vi "ShopTable.vi"(4 "食品信息":cluster{"ID":dbl, "食品名称":string, "价格":dbl}, 6 "枚举":enum16{"保存", "获取", "清空", "插入", "删除", "查询"}(ring)) -> (0 "Exist?":bool, 2 "食品信息 2":cluster{"ID":dbl, "食品名称":string, "价格":dbl}, 3 "数组":cluster{"ID":dbl, "食品名称":string, "价格":dbl}[](array[cluster]))   [LabVIEW 2013, in "InfoTable.lvclass"]
uses:
  InfoTable.lvclass
  FoodBase.lvclass
panel:
  in  "第一次？":bool
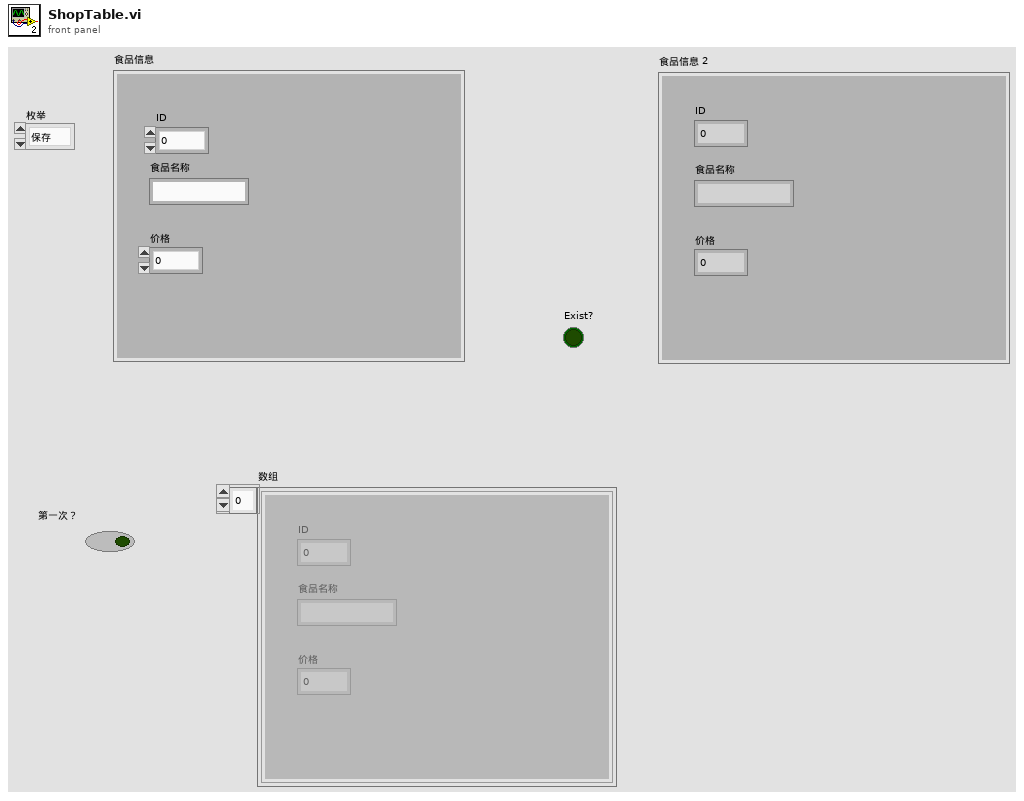
[diagram p1: front panel]
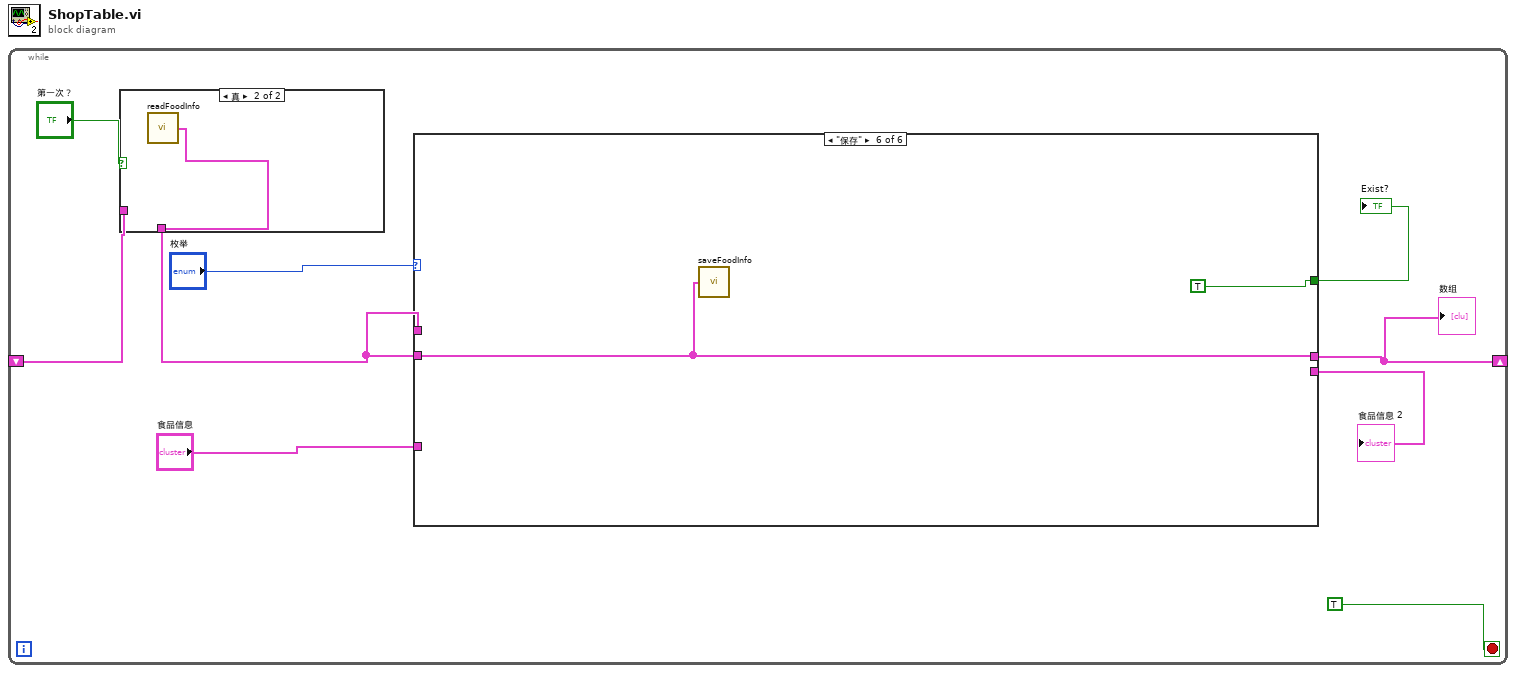
[diagram p0: block diagram]
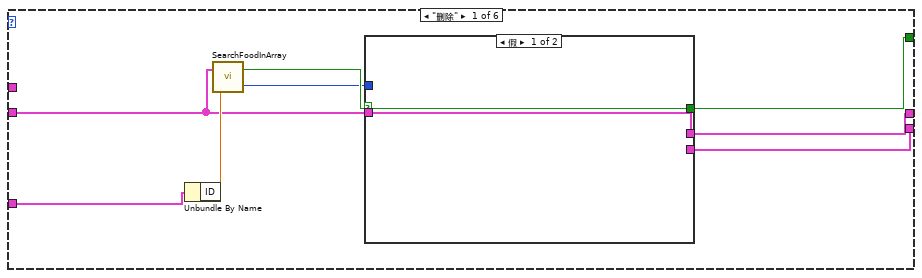
[diagram p3: hidden frame]
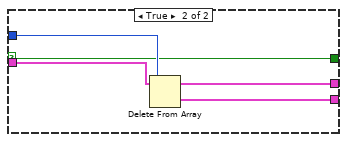
[diagram p4: hidden frame]
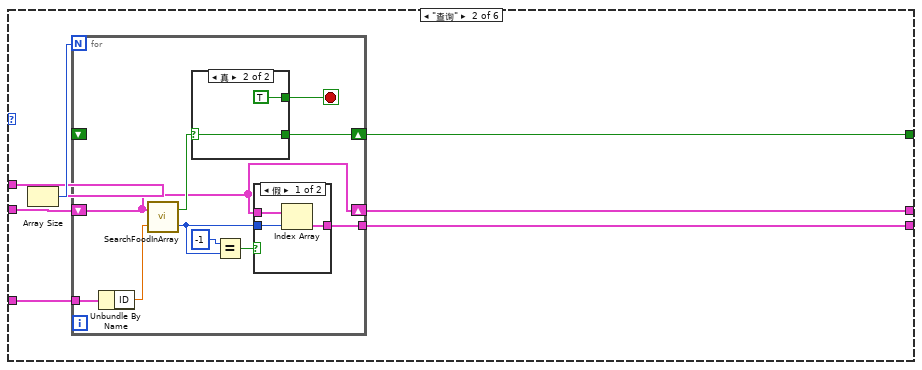
[diagram p5: hidden frame]
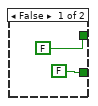
[diagram p7: hidden frame]
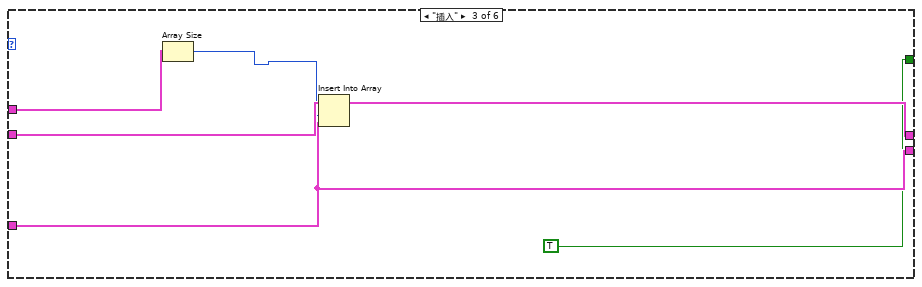
[diagram p8: hidden frame]
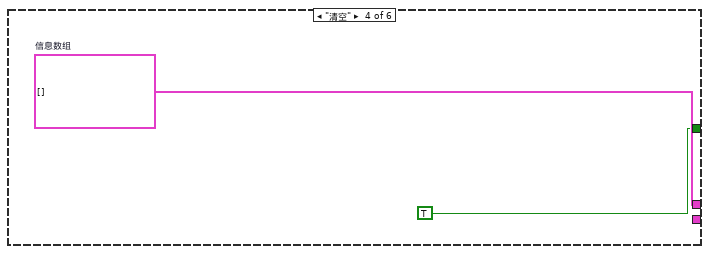
[diagram p9: hidden frame]
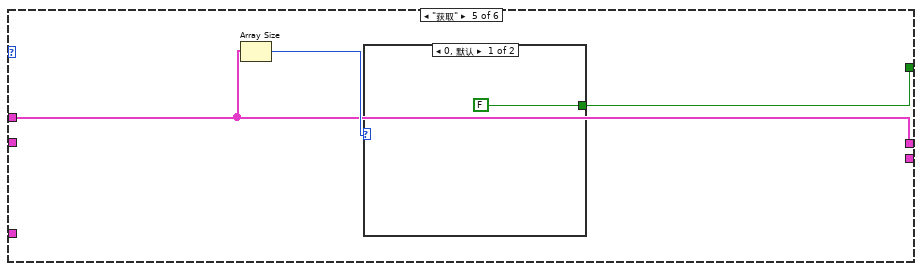
[diagram p10: hidden frame]
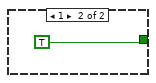
[diagram p11: hidden frame]
diagram:
  n1 = while {
    shift-right: [w2] -> _
    shift-left: _ -> [w4]
    stop <- TRUE stop-if-true
    n2 = case shown="真" "第一次？" {
      tunnel: [w10 w11] -> w5
      tunnel: w4 -> [w10 _]
      frame False {
      }
      frame True {
        n3 = call "readFoodInfo.vi"() -> ("数组"=w11:cluster{"ID":dbl, "食品名称":string, "价格":dbl}[])
      }
    }
    n4 = case shown="\"保存\"" "枚举" {
      tunnel: w5 -> [_ w32 w56 _ w59 _]
      tunnel: w5 -> [w16 w31 w55 _ _ w65]
      tunnel: [w13 w30 TRUE TRUE w60 TRUE] -> w7
      tunnel: [w12 w29 w53 _ _ _] -> w8
      tunnel: "食品信息" -> [w19 w28 w53 _ _ _]
      tunnel: [w14 w27 w54 w58 w59 w65] -> w2
      frame "删除" {
        n5 = Unbundle By Name(w19) -> ("ID"=w18:dbl)
        n6 = call "SearchFoodInArray.vi"("ID"=w18, "信息数组"=w16) -> ("Found Index"=w15:i32, "Exist?"=w17:bool)
        n7 = case shown="假" w17 {
          selector: w17 -> [w20 w22]
          tunnel: w16 -> [w21 w26]
          tunnel: w15 -> [_ w25]
          tunnel: [_ w24] -> w12
          tunnel: [w21 w23] -> w14
          tunnel: [w20 w22] -> w13
          frame False {
          }
          frame True {
            n8 = Delete From Array(array=w26, index=w25) -> (deleted portion=w24:cluster{"ID":dbl, "食品名称":string, "价格":dbl}, array with subset deleted=w23:cluster{"ID":dbl, "食品名称":string, "价格":dbl}[])  [unwired: 1 in]
          }
        }
      }
      frame "查询" {
        n9 = Array Size(array=w32) -> (size(s)=w33:i32)
        n10 = for {
          N: w33 -> [_]
          shift-right: [w36] -> w27
          shift-left: w31 -> [w36]
          shift-right: [w41] -> w30
          shift-left: _ -> [_]
          tunnel: [w35] -> w29
          tunnel: w28 -> [w34]
          stop <- w40 stop-if-true
          n11 = Unbundle By Name(w34) -> ("ID"=w43:dbl)
          n12 = call "SearchFoodInArray.vi"("ID"=w43, "信息数组"=w36) -> ("Found Index"=w37:i32, "Exist?"=w42:bool)
          n13 = case shown="真" w42 {
            selector: w42 -> [_ w50]
            tunnel: [FALSE w50] -> w41
            tunnel: [FALSE TRUE] -> w40
            frame False {
            }
            frame True {
            }
          }
          n14 = Equal?(x=-1, y=w37) -> (x = y?=w38:bool)
          n15 = case shown="假" w38 {
            tunnel: w37 -> [w46 _]
            tunnel: w36 -> [w45 _]
            tunnel: [w44 _] -> w35
            frame False {
              n16 = Index Array(array=w45, index=w46) -> (element=w44:cluster{"ID":dbl, "食品名称":string, "价格":dbl})
            }
            frame True {
            }
          }
        }
      }
      frame "插入" {
        n17 = Array Size(array=w56) -> (size(s)=w51:i32)
        n18 = Insert Into Array(array=w55, index=w51, new element=w53) -> (w54:cluster{"ID":dbl, "食品名称":string, "价格":dbl}[])
      }
      frame "清空" {
        w58 = cluster{"ID":dbl, "食品名称":string, "价格":dbl}[] []  # 信息数组
      }
      frame "获取" {
        n19 = Array Size(array=w59) -> (size(s)=w61:i32)
        n20 = case shown="0, 默认" w61 {
          tunnel: [FALSE TRUE] -> w60
          frame 0, Default {
          }
          frame 1 {
          }
        }
      }
      frame "保存" {
        n21 = call "saveFoodInfo.vi"("数组"=w65) -> ()
      }
    }
    "食品信息 2" <- w8
    "Exist?" <- w7
    "数组" <- w2
  }
